vi "Get Total Duration (s).vi"(8 "error in (no error)":errorcluster, 11 "SongLibrary in":refnum<class "SongLibrary.lvclass">) -> (0 "error out":errorcluster, 2 "Duration (s)":T1 format="%<%M:%S>T", 3 "SongLibrary out":refnum<class "SongLibrary.lvclass">)   [LabVIEW 2015, in "SongLibrary.lvclass"]
uses:
  SongLibrary.lvclass
  Song/Song Duration.ctl
  MusicElementLibrary.lvclass/MusicElementLibrary.ctl
  Song/Song.lvclass/Song.ctl
  Song/Read Duration (s).vi
  MusicElement.lvclass
  Song/Song.lvclass
  MusicElementLibrary.lvclass
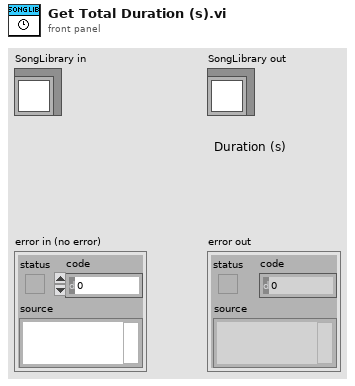
[diagram p1: front panel]
types:
  T1 = typedef "Song.lvclass/Song Duration.ctl" = timestamp
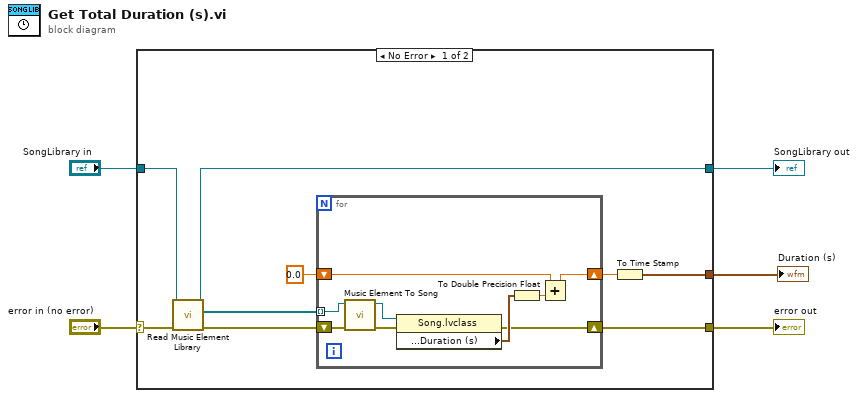
[diagram p0: block diagram]
diagram:
  n1 = case shown="No Error" "error in (no error)" {
    selector: "error in (no error)" -> [w10 w25]
    tunnel: [w12 w25] -> w4
    tunnel: [w7 w24] -> w2
    tunnel: "SongLibrary in" -> [w9 w24]
    tunnel: [w11 _] -> w1
    frame No Error {
      n2 = call "Read Music Element Library.vi"("error in (no error)"=w10, "MusicElementLibrary in"=w9) -> ("error out"=w8:errorcluster, "Music Element Library"=w6:refnum<class "MusicElement.lvclass">[], "MusicElementLibrary out"=w7:refnum<class "SongLibrary.lvclass">)  [unwired: 7 in]
      n3 = for {
        shift-right: [w19] -> w12
        shift-left: w8 -> [w18]
        shift-right: [w21] -> w13
        shift-left: 0.0 -> [w20]
        tunnel: w6 -> [w16] mode=indexing
        n4 = call "Music Element To Song.vi"("error in (no error)"=w18, "MusicElement"=w16) -> ("error out"=w17:errorcluster, "Song out"=w15:refnum<class "Song.lvclass">)  [unwired: 8 in]
        n5 = property class="Song.lvclass"(reference=w15, error in=w17) -> (error out=w19:errorcluster, "API:Data Member Accessors:Duration (s)"=w23:T1)  [unwired: 1 out]
        n6 = To Double Precision Float(number=w23) -> (double precision float=w22:dbl)
        n7 = Add(x=w20, y=w22) -> (x+y=w21:dbl)
      }
      n8 = To Time Stamp(1:w13) -> (0:w11:timestamp)
    }
    frame Error {
    }
  }
  "error out" <- w4
  "SongLibrary out" <- w2
  "Duration (s)" <- w1
